vi "TestingSound.vi"() -> ()   [LabVIEW 2009]
panel:
  in  "Play?":bool
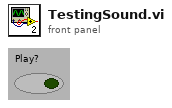
[diagram p1: front panel]
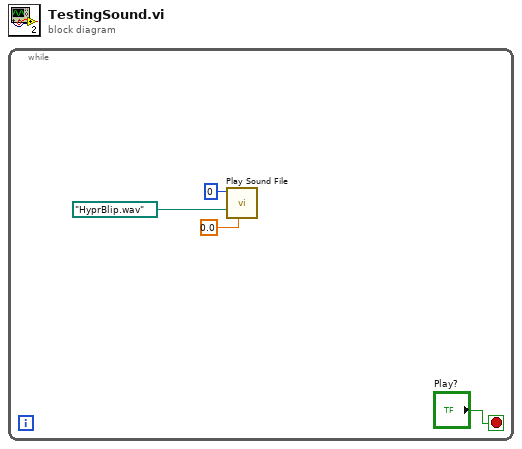
[diagram p0: block diagram]
diagram:
  n1 = while {
    stop <- "Play?" stop-if-true
    n2 = call <vilib>:"Play Sound File.vi"("timeout (sec)"=0.0, "path"=path "HyprBlip.wav", "device ID"=u32 0) -> ()  [unwired: 7 in, 2 out]
  }
